vi "HapticSTM_flt.vi"() -> ()   [LabVIEW 2019]
uses:
  <vilib>/sound2/lvsound2.llb/Sampling Mode.ctl
  <vilib>/sound2/lvsound2.llb/Sound Data Format.ctl
  SubVIs/GlobalClicksHeight_flt.vi
  <vilib>/Utility/file.llb/Read Delimited Spreadsheet (DBL).vi
  <vilib>/sound2/lvsound2.llb/Sound Output Set Volume (Single).vi
  <vilib>/sound2/lvsound2.llb/Sound Output Write (DBL Single).vi
  <userlib>/HapticSTM/HapticSTM.lvlib
panel:
  in  "Sensitivity":dbl=1.0 format="%.1f"
  in  "Volume":dbl(slide)=50.0 scale=0.0..100.0
  in  "Device ID":u32
  in  "Planing?":bool
  in  "Setpoint (pA)":dbl=100.0
  in  "Plunge Depth (pA)":dbl=280.0 format="%.1f"
  out "Button":bool
  out "Setpoint (pA)":dbl
  in  "Maximum (pA)":dbl=9000.0
  out "Filtered Current (pA)":dbl format="%.1f"
  out "Current (pA)":dbl format="%.1f"
  out "Oy":dbl
  out "Ox":dbl
  out "W":dbl
  out "H":dbl
  out "Z Write":dbl format="%^.1e"
  out "Z Read":dbl format="%^#.1e"
  out "Vy":dbl format="%.1f"
  out "Vz":dbl format="%.1f"
  out "Vx":dbl format="%.1f"
  out "Fy":dbl format="%.1f"
  out "Fz":dbl format="%.1f"
  out "Fx":dbl format="%.1f"
  out "phi":dbl format="%.1f"
  out "psi":dbl format="%.1f"
  out "theta":dbl format="%.1f"
  out "x":dbl format="%.1f"
  out "y":dbl format="%.1f"
  out "z":dbl format="%0.1f"
  out "Height":dbl format="%^.1e"
  in  "Hardness":dbl=1.0 format="%.1f"
  in  "Mode":u16(ring) items=["Log w/ Exp Z", "Log w/ Lin Z"]
  in  "Reset Clicks":bool
  out "Clicks":i32
  in  "STOP":bool
  in  "START":bool
  out "Seq":i32
  out "SeqString":string
  out "Raw and Scaled Z Positions":cluster{dbl, "Y":dbl}(graph)
  out "Scaled Force and Current":cluster{dbl, "Filtered x":dbl, dbl}(graph)
  in  "Tab Control":T1(tab)
  # "temporary"
  # "No"
  # "Yes"
  # "Nanonis"
  # "Current"
  # "Frame"
  # "Z Controller"
  # "Haptic Pen"
  # "Position"
  # "Force"
  # "Angles"
  # "Velocity"
  # "Surface"
  # "Clicks"
  # "Haptic STM Controller 3000"
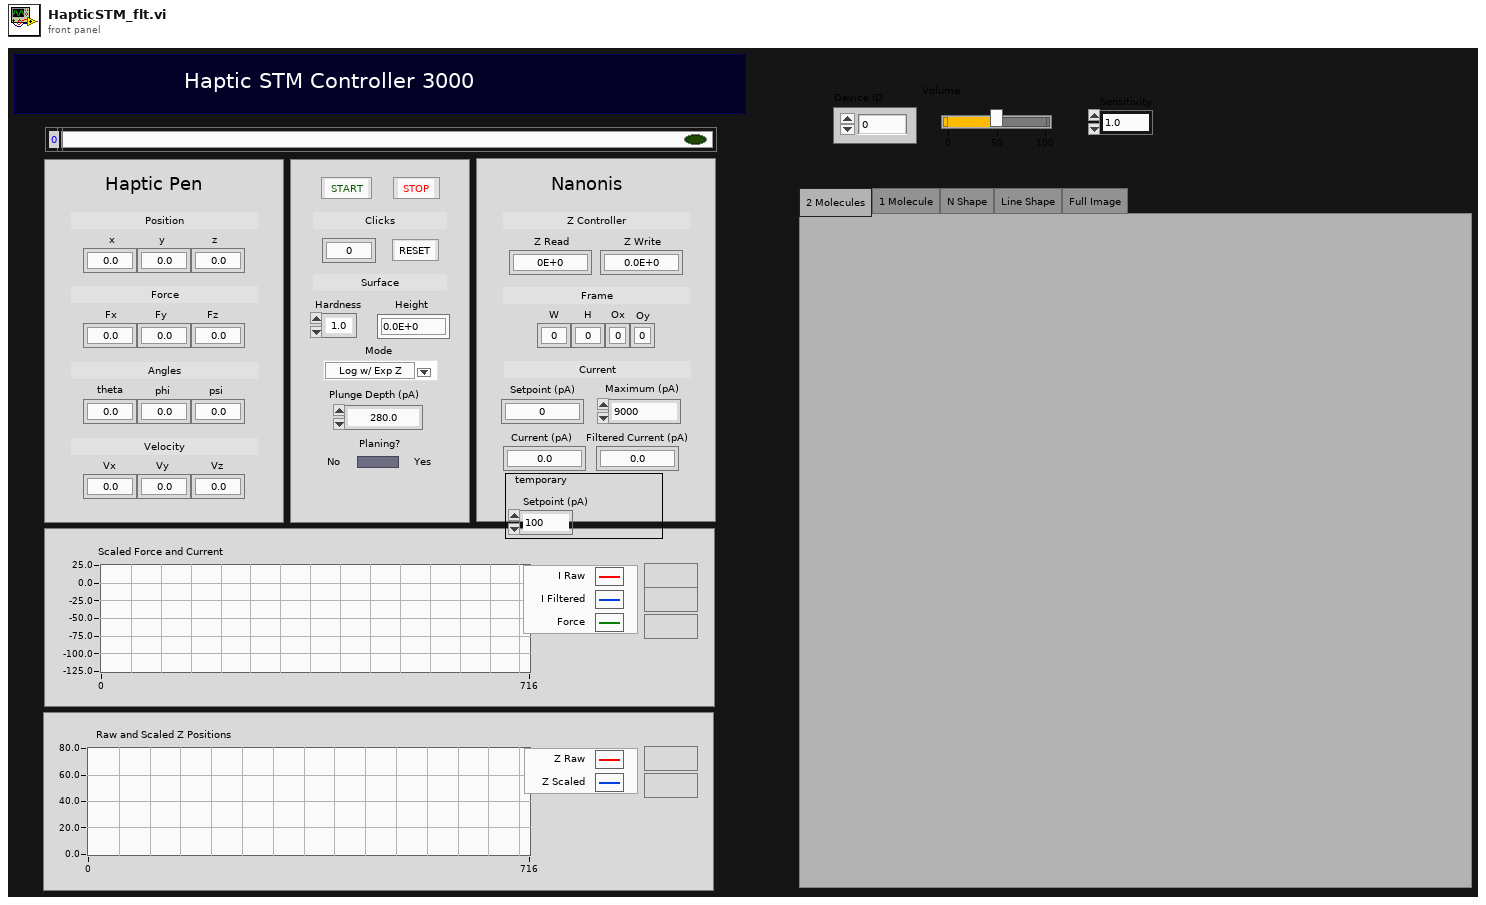
[diagram p1: front panel]
types:
  T1 = enum32{"2 Molecules", "1 Molecule", "N Shape", "Line Shape", "Full Image"}
  T2 = typedef "Sound Data Format.ctl" = cluster{"sample rate (S/s)":dbl, "number of channels":i32, "bits per sample":i32}
  T3 = typedef "Sampling Mode.ctl" = i32
  T4 = typedef "Sound Output Task ID.ctl" = u32
  T5 = cluster{"Current Out (pA)":dbl, "Filtered Current (pA)":dbl, dbl}
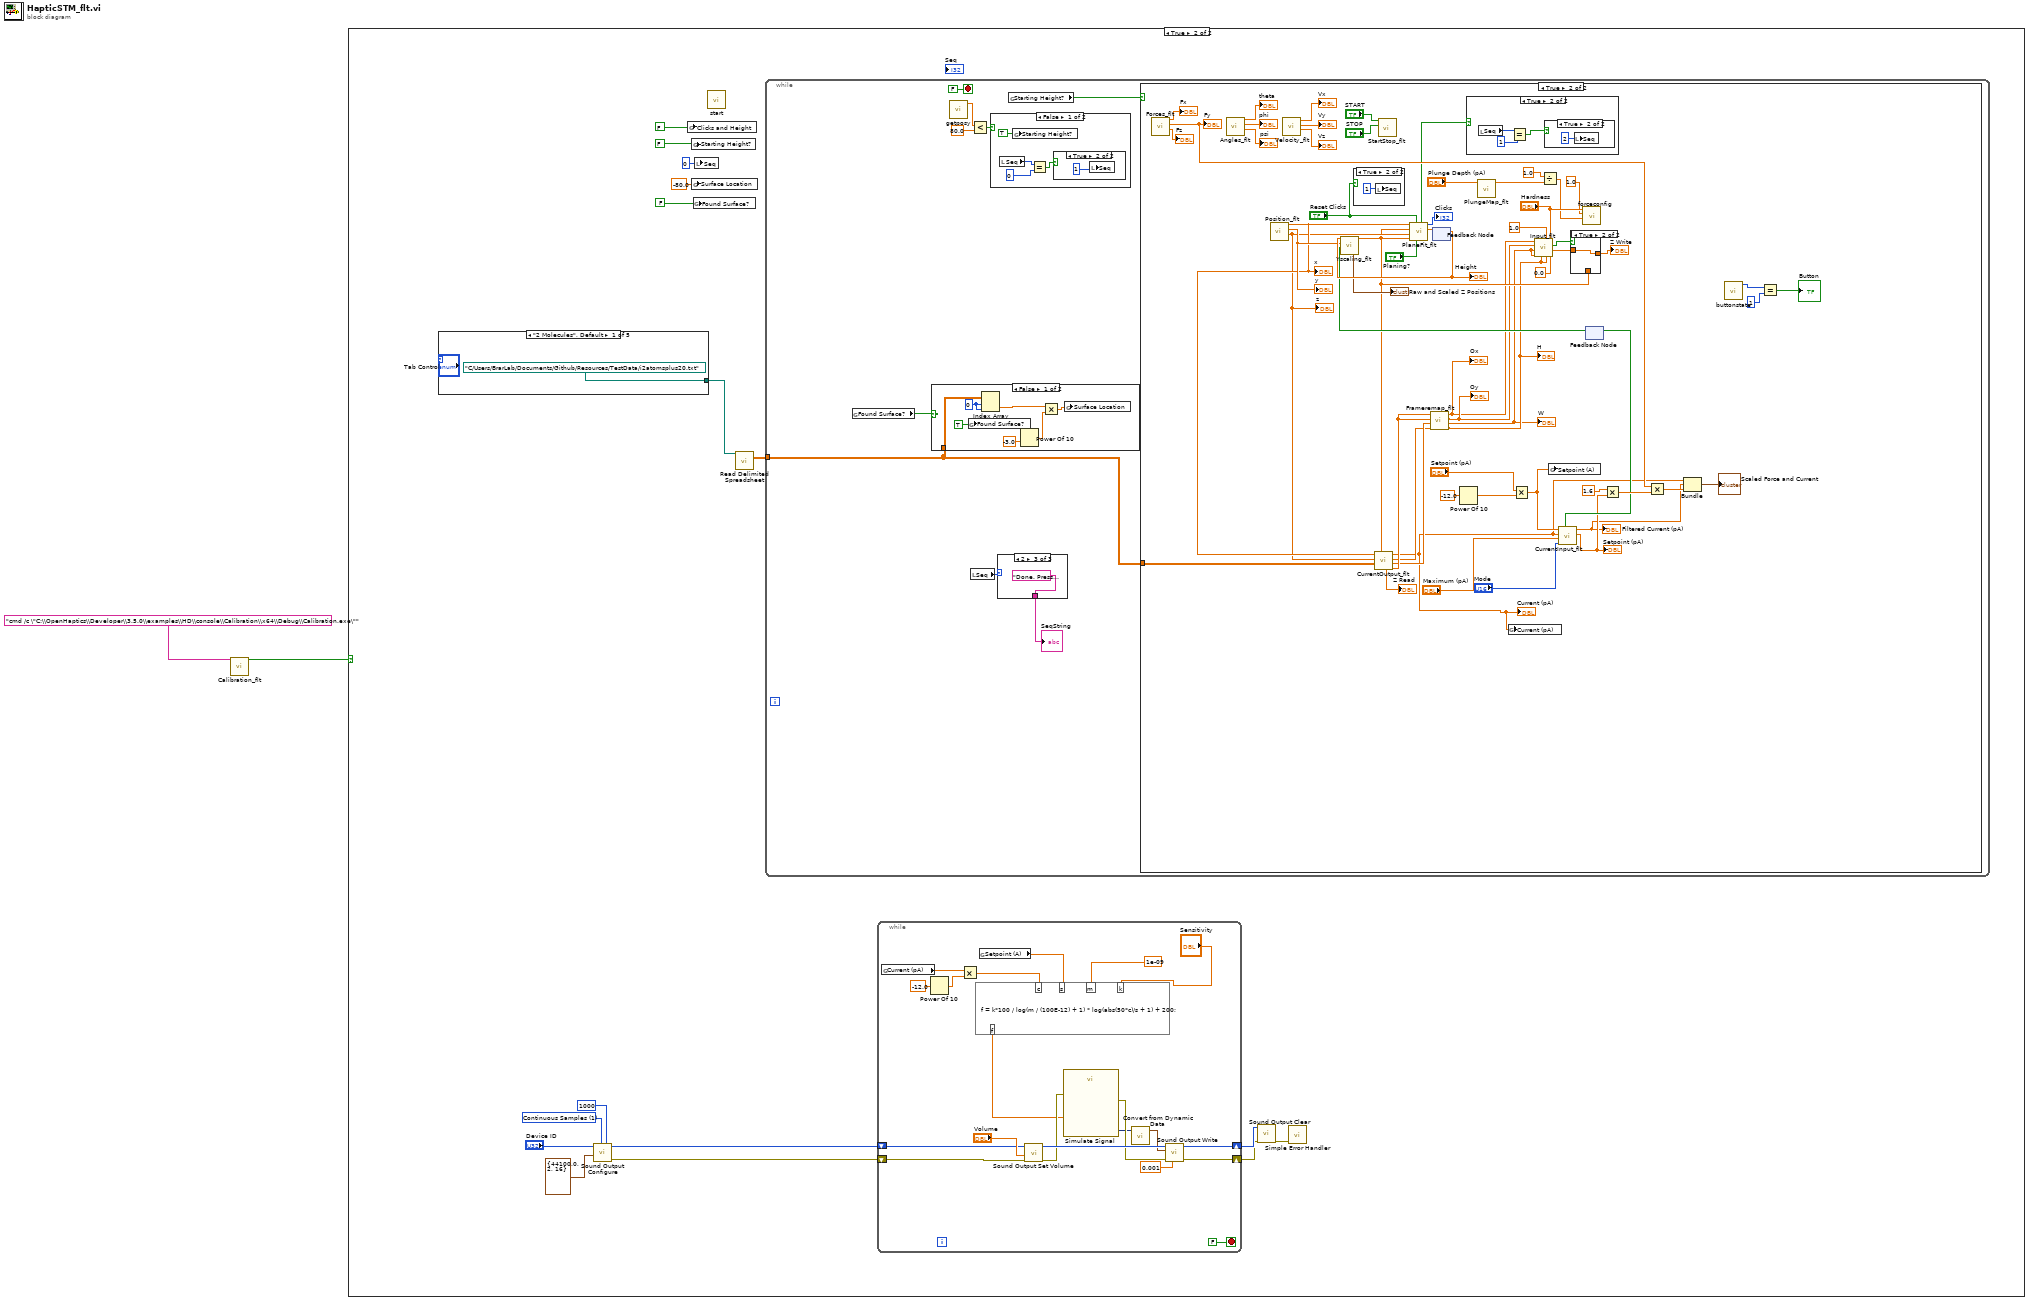
[diagram p0: block diagram]
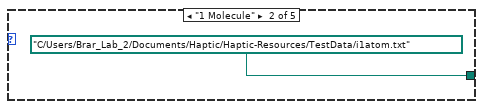
[diagram p3: hidden frame]
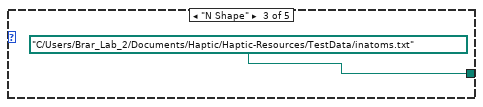
[diagram p4: hidden frame]
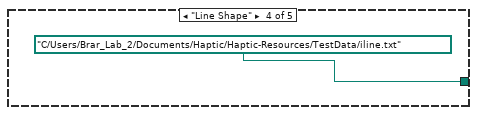
[diagram p5: hidden frame]
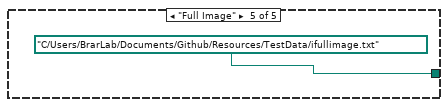
[diagram p6: hidden frame]
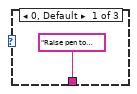
[diagram p8: hidden frame]
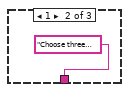
[diagram p9: hidden frame]
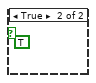
[diagram p11: hidden frame]
diagram:
  n1 = call "Calibration_flt.vi"("command line"="cmd /c \"C:\\OpenHaptics\\Developer\\3.5.0\\examples\\HD\\console\\Calibration\\x64\\Debug\\Calibration.exe\"") -> ("Calibration Complete?"=w2:bool)  [unwired: 10 in]
  n2 = case shown="True" w2 {
    frame False {
    }
    frame True {
      w10 = T3 1 items=["Finite Samples", "Continuous Samples"] ("sample mode")
      n3 = case shown="\"2 Molecules\", Default" "Tab Control" {
        tunnel: [path "C:/Users/BrarLab/Documents/Github/Resources/TestData/i2atomsplus20.txt" ("file path (dialog if empty)") path "C:/Users/Brar_Lab_2/Documents/Haptic/Haptic-Resources/TestData/i1atom.txt" ("file path (dialog if empty)") path "C:/Users/Brar_Lab_2/Documents/Haptic/Haptic-Resources/TestData/inatoms.txt" ("file path (dialog if empty)") path "C:/Users/Brar_Lab_2/Documents/Haptic/Haptic-Resources/TestData/iline.txt" ("file path (dialog if empty)") path "C:/Users/BrarLab/Documents/Github/Resources/TestData/ifullimage.txt" ("file path (dialog if empty)")] -> w14
        frame "2 Molecules", Default {
        }
        frame "1 Molecule" {
        }
        frame "N Shape" {
        }
        frame "Line Shape" {
        }
        frame "Full Image" {
        }
      }
      n4 = call <vilib>:"Sound Output Configure.vi"("number of samples/ch"=1000 ("Number of Samples/ch"), "sample mode"=w10, "sound format"=T2 {"sample rate (S/s)"=44100.0, "number of channels"=2, "bits per sample"=16} ("Sound Format"), "device ID"="Device ID") -> ("error out"=w6:errorcluster, "task ID"=w7:T4)  [unwired: 6 in]
      n5 = global write "GlobalClicksHeight_flt.vi" "Clicks and Height"(FALSE ("Clicks and Height")) -> ()
      n6 = global write "GlobalClicksHeight_flt.vi" "Starting Height?"(FALSE ("Clicks and Height")) -> ()
      n7 = global write "GlobalClicksHeight_flt.vi" "Surface Location"(-80.0 ("Surface Location")) -> ()
      n8 = global write "GlobalClicksHeight_flt.vi" "Found Surface?"(FALSE ("Clicks and Height")) -> ()
      n9 = local write "Seq"(0 ("Seq")) -> ()
      n10 = call <userlib>:"start.vi"() -> ()  [unwired: 11 in, 1 out]
      n11 = call-poly <vilib>:"Read Delimited Spreadsheet.vi"("file path (dialog if empty)"=w14) -> ("all rows"=w19:dbl[][])  [unwired: 9 in, 5 out]
      n12 = while {
        tunnel: w19 -> [w46]
        stop <- FALSE stop-if-true
        n13 = global read "GlobalClicksHeight_flt.vi" "Found Surface?"() -> (w45:bool)
        n14 = case shown="False" w45 {
          tunnel: w46 -> [w58 _]
          frame False {
            w60 = 0 ("index (row)")
            n15 = global write "GlobalClicksHeight_flt.vi" "Found Surface?"(TRUE ("Found Surface?")) -> ()
            n16 = Index Array(array=w58, index (row)=w60, index (col)=w60) -> (element=w57:dbl)
            n17 = Power Of 10(x=-3.0) -> (10^x=w55:dbl)
            n18 = Multiply(x=w57, y=w55) -> (x*y=w56:dbl)
            n19 = global write "GlobalClicksHeight_flt.vi" "Surface Location"(w56) -> ()
          }
          frame True {
          }
        }
        n20 = call <userlib>:"getposy.vi"() -> ("function return"=w53:dbl)  [unwired: 11 in]
        n21 = local read "Seq"() -> (w48:i32)
        n22 = Less?(x=w53, y=80.0) -> (x < y?=w51:bool)
        n23 = case shown="False" w51 {
          frame False {
            n24 = local read "Seq"() -> (w66:i32)
            n25 = global write "GlobalClicksHeight_flt.vi" "Starting Height?"(TRUE ("Starting Height?")) -> ()
            n26 = Equal?(x=w66, y=0) -> (x = y?=w64:bool)
            n27 = case shown="True" w64 {
              frame False {
              }
              frame True {
                n28 = local write "Seq"(1 ("Seq")) -> ()
              }
            }
          }
          frame True {
            (unwired) TRUE ("Clicks and Height")
          }
        }
        n29 = case shown="2" w48 {
          tunnel: ["Raise pen to begin." "Choose three points, then raise the arm to plane." "Done. Press 'STOP' to stop at anytime."] -> w47
          frame 0, Default {
          }
          frame 1 {
          }
          frame 2 {
          }
        }
        "SeqString" <- w47
        n30 = global read "GlobalClicksHeight_flt.vi" "Starting Height?"() -> (w50:bool)
        n31 = case shown="True" w50 {
          tunnel: w46 -> [_ w100]
          frame False {
          }
          frame True {
            n32 = call "Forces_flt.vi"() -> ("Fz"=→"Fz":dbl, "Fy"=w110:dbl, "Fx"=→"Fx":dbl)  [unwired: 9 in]
            "Fy" <- w110
            n33 = call "Angles_flt.vi"() -> ("psi"=→"psi":dbl, "phi"=→"phi":dbl, "theta"=→"theta":dbl)  [unwired: 9 in]
            n34 = call "Position_flt.vi"() -> ("Z"=w101:dbl, "Y"=w106:dbl, "X"=w102:dbl)  [unwired: 9 in]
            "x" <- w102
            "y" <- w106
            "z" <- w101
            n35 = call "Velocity_flt.vi"() -> ("VZ"=→"Vz":dbl, "VY"=→"Vy":dbl, "VX"=→"Vx":dbl)  [unwired: 9 in]
            n36 = case shown="True" "Reset Clicks" {
              frame False {
              }
              frame True {
                n37 = local write "Seq"(1 ("Seq")) -> ()
              }
            }
            n38 = call "StartStop_flt.vi"("STOP"="STOP", "START"="START") -> ()  [unwired: 10 in]
            n39 = feedback #1() -> (w116:dbl)  [unwired: 1 in]
            "Height" <- w116
            n40 = Power Of 10(x=-12.0) -> (10^x=w115:dbl)
            n41 = call "PlungeMap_flt.vi"("Input (pA)"="Plunge Depth (pA)") -> ("output"=w69:dbl)  [unwired: 10 in]
            n42 = Multiply(x="Setpoint (pA)", y=w115) -> (x*y=w77:dbl)
            n43 = Divide(x=1.0, y=w69) -> (x/y=w87:dbl)
            n44 = global write "GlobalClicksHeight_flt.vi" "Setpoint (A)"(w77) -> ()
            n45 = call <userlib>:"forceconfig.vi"("c"=w87, "b"=1.0, "a"="Hardness") -> ()  [unwired: 9 in]
            n46 = feedback #2() -> (w112:bool)  [unwired: 1 in]
            n47 = call "Yscaling_flt.vi"("Current Maxed?"=w112, "Y"=w106, "Plane Height"=w116) -> ("y scaled"=w89:dbl, "Zpos Graph (nm)"=→"Raw and Scaled Z Positions":cluster{dbl, "function return":dbl})  [unwired: 7 in]
            n48 = call "CurrentOutput_flt.vi"("y scaled"=w89, "array"=w100, "Z Input"=w101, "X Input"=w102) -> ("Origin"=w85:dbl, "FW"=w84:dbl, "FH"=w83:dbl, "Current Out (pA)"=w72:dbl, "Zread"=→"Z Read":dbl)  [unwired: 3 in]
            "Current (pA)" <- w72
            n49 = call "PlaneFit_flt.vi"("Planing y/n?"="Planing?", "Reset Clicks"="Reset Clicks", "Y PEN"=w89, "Z"=w101, "Nano Z"=w89, "X"=w102) -> ("Plane Height (m)"=w117:dbl, "Clicks"=→"Clicks":i32, "Planing Done?"=w96:bool)  [unwired: 3 in]
            n50 = call "Frameremap_flt.vi"("FH"=w83, "FW"=w84, "FO Z"=w85, "FO X"=w85) -> ("FH"=w82:dbl, "FW"=w81:dbl, "Z Origin"=w80:dbl, "X Origin"=w79:dbl)  [unwired: 4 in]
            "H" <- w82
            "W" <- w81
            "Ox" <- w79
            "Oy" <- w80
            n51 = feedback-in #1(w117) -> ()
            n52 = case shown="True" w96 {
              frame False {
              }
              frame True {
                n53 = local read "Seq"() -> (w134:i32)
                n54 = Equal?(x=w134, y=1) -> (x = y?=w132:bool)
                n55 = case shown="True" w132 {
                  frame False {
                  }
                  frame True {
                    n56 = local write "Seq"(2 ("Seq")) -> ()
                  }
                }
              }
            }
            n57 = global write "GlobalClicksHeight_flt.vi" "Current (pA)"(w72) -> ()
            n58 = call "Input_flt.vi"("Current * 10^input"=0.0, "Sensitivity"="Hardness", "Scopez"=w82, "Drag"=1.0, "FH"=w82, "FW"=w81, "Scopex"=w81, "Z origin"=w80, "X origin"=w79) -> ("Scaled Current"=w90:dbl, "feedback"=w92:bool)  [unwired: 1 in]
            n59 = call "CurrentInput_flt.vi"("Mode"="Mode", "Maximum (pA)"="Maximum (pA)", "Current (pA)"=w72, "Setpoint (A)"=w77) -> ("Setpoint (pA)"=w73:dbl, "Filtered Current (pA)"=w71:dbl, "Current Maxed?"=w74:bool)  [unwired: 5 in]
            "Filtered Current (pA)" <- w71
            "Setpoint (pA)" <- w73
            n60 = case shown="True" w92 {
              tunnel: [w129 w130] -> w91
              tunnel: w90 -> [_ w130]
              tunnel: w89 -> [w129 _]
              frame False {
              }
              frame True {
              }
            }
            "Z Write" <- w91
            n61 = feedback-in #2(w74) -> ()
            n62 = Multiply(x=1.6 ("y"), y=w73) -> (x*y=w107:dbl)
            n63 = Multiply(x=w110, y=w107) -> (x*y=w109:dbl)
            n64 = Bundle("Current Out (pA)"=w72, "Filtered Current (pA)"=w71, w109) -> (→"Scaled Force and Current":T5)  [unwired: 1 in]
            n65 = call <userlib>:"buttonstate.vi"() -> ("function return"=w105:i32)  [unwired: 11 in]
            n66 = Equal?(x=w105, y=1) -> (x = y?=→"Button":bool)
          }
        }
      }
      n67 = while {
        shift-right: [w31] -> w5
        shift-left: w7 -> [w33]
        shift-right: [w30] -> w4
        shift-left: w6 -> [w32]
        stop <- FALSE stop-if-true
        n68 = global read "GlobalClicksHeight_flt.vi" "Current (pA)"() -> (w22:dbl)
        n69 = Power Of 10(x=-12.0) -> (10^x=w24:dbl)
        n70 = Multiply(x=w22, y=w24) -> (x*y=w21:dbl)
        n71 = global read "GlobalClicksHeight_flt.vi" "Setpoint (A)"() -> (w26:dbl)
        n72 = formula code="f = k*100 / log(m / (100E-12) + 1) * log(abs(50*c)/s + 1) + 200;"("c"=w21, "m"=1e-09 ("input variable"), "s"=w26, "k"="Sensitivity") -> ("f"=w25:dbl)
        n73 = call-poly <vilib>:"Sound Output Set Volume.vi"("error in (no error)"=w32, "volume"="Volume", "task ID"=w33) -> ("error out"=w36:errorcluster, "task ID out"=w39:T4)  [unwired: 7 in]
        n74 = call "Simulate Signal"("Frequency"=w25, "error in (no error)"=w36) -> ("Sine"=w34:dynamicdata, "error out"=w35:errorcluster)  [unwired: 12 in]
        n75 = call "Convert from Dynamic Data"("Dynamic Data Type"=w34) -> ("Waveform"=w37:waveform(dbl))  [unwired: 3 in]
        n76 = call-poly <vilib>:"Sound Output Write.vi"("timeout (sec)"=0.001, "error in (no error)"=w35, "data"=w37, "task ID"=w39) -> ("error out"=w30:errorcluster, "task ID out"=w31:T4)  [unwired: 6 in]
      }
      n77 = call <vilib>:"Sound Output Clear.vi"("error in (no error)"=w4, "task ID"=w5) -> ("error out"=w9:errorcluster)  [unwired: 9 in]
      n78 = call <vilib>:"Simple Error Handler.vi"("error in (no error)"=w9) -> ()  [unwired: 4 in, 5 out]
    }
  }
